vi "Debug Path.vi"() -> (0 "Debug Path":path)   [LabVIEW 2020, in "G-Unicode.lvlib"]
uses:
  G-Unicode.lvlib
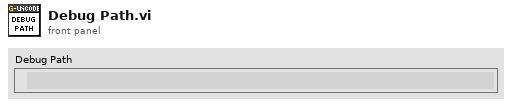
[diagram p1: front panel]
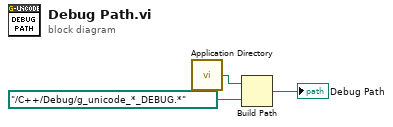
[diagram p0: block diagram]
diagram:
  n1 = call <vilib>:"Application Directory.vi"() -> ("Application Directory"=w3:path)
  n2 = Build Path(base path=w3, name or relative path=path "../C++/Debug/g_unicode_*_DEBUG.*") -> (appended path=→"Debug Path":path)
